vi "Build.vi"   [LabVIEW 2017]
doc: "Builds all of the build specifications defined in this project."
uses:
  <vilib>/AppBuilder/AB_API_Simple/Build (path).vi
  <vilib>/AppBuilder/AB_API_Simple/NI_App_Builder_API.lvlib
panel:
  # "Overview: Builds all Source Distribution specifications for this project\nRequirements: LabVIEW\nInstructions: Run this VI.\n\nThis VI builds all of the build specifications for this project. Any version of LabVIEW that supports projects and the Application Builder API can be used."
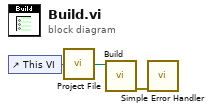
[diagram p0: block diagram]
diagram:
  n1 = control-ref of="This VI"() -> (w1:refnum<vi>)
  n2 = call "Project File.vi"("VI"=w1) -> ("Project File"=w2:path)
  n3 = call-poly <vilib>:"Build.vi"("Path to project"=w2) -> ("error out"=w3:errorcluster)  [unwired: 9 in, 1 out]
  n4 = call <vilib>:"Simple Error Handler.vi"("error in (no error)"=w3) -> ()  [unwired: 4 in, 5 out]
